vi "Ref_2_R.vi"(0 "Control  Ch 3":refnum<vi>, 1 "Control  Ch 4":refnum<vi>, 2 "Control  Ch 5":refnum<vi>, 3 "Init_F":bool=TRUE, 4 "Control  Ch 6":refnum<vi>, 5 "Control  Ch 7":refnum<vi>, 6 "Control  Ch 8":refnum<vi>, 7 "error in":errorcluster, 8 "Control  Ch 2":refnum<vi>, 9 "Control  Ch 10":refnum<vi>, 10 "Control  Ch 1":refnum<vi>, 11 "Control  Ch 11":refnum<vi>, 12 "Control  Ch 9":refnum<vi>, 13 "Control  Ch 12":refnum<vi>) -> (15 "Control  Ch 12 out":refnum<vi>, 16 "Control  Ch 10 out":refnum<vi>, 17 "Control  Ch 1 out":refnum<vi>, 18 "Control  Ch 9 out":refnum<vi>, 19 "Control  Ch 2 out":refnum<vi>, 20 "Control  Ch 11 out":refnum<vi>, 21 "Control  Ch 8 out":refnum<vi>, 22 "Control  Ch 7 out":refnum<vi>, 23 "Control  Ch 6 out":refnum<vi>, 24 "Control  Ch 5 out":refnum<vi>, 25 "Control  Ch 4 out":refnum<vi>, 26 "Control  Ch 3 out":refnum<vi>, 27 "error out":errorcluster)   [LabVIEW 2017]
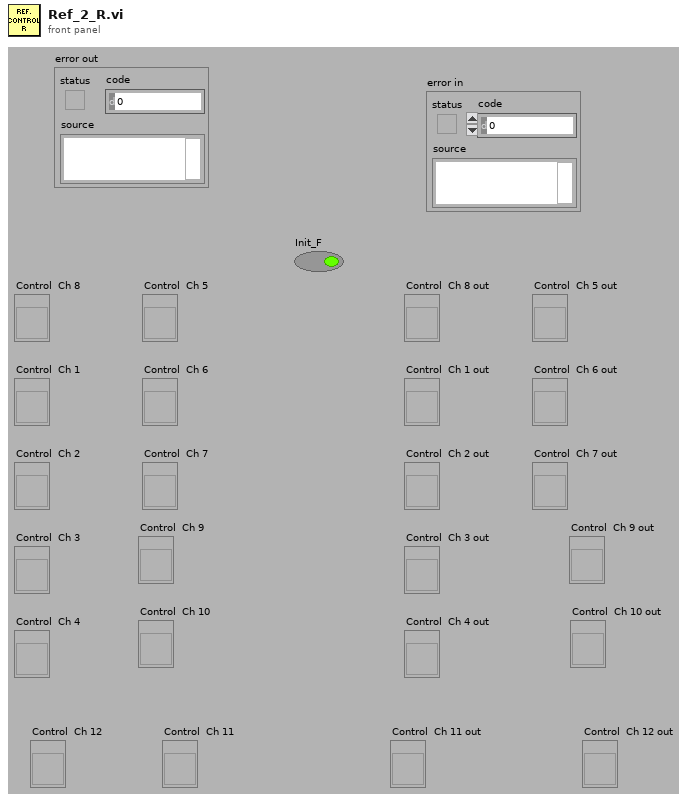
[diagram p1: front panel]
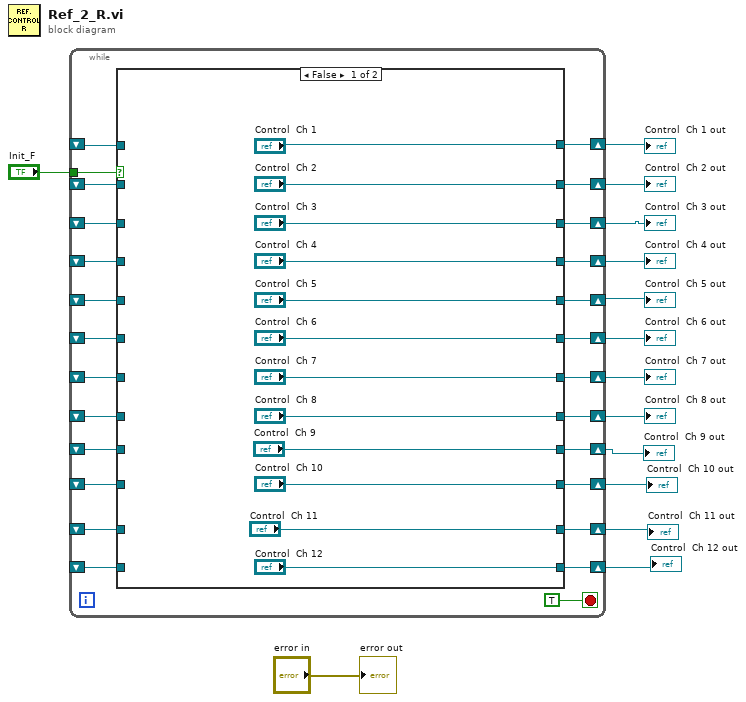
[diagram p0: block diagram]
diagram:
  n1 = while {
    shift-right: [w39] -> w12
    shift-left: _ -> [w38]
    tunnel: "Init_F" -> [w37]
    shift-right: [w36] -> w11
    shift-left: _ -> [w29]
    shift-right: [w35] -> w8
    shift-left: _ -> [w28]
    shift-right: [w34] -> w10
    shift-left: _ -> [w23]
    shift-right: [w33] -> w9
    shift-left: _ -> [w27]
    shift-right: [w32] -> w7
    shift-left: _ -> [w26]
    shift-right: [w31] -> w6
    shift-left: _ -> [w25]
    shift-right: [w30] -> w5
    shift-left: _ -> [w24]
    shift-right: [w22] -> w4
    shift-left: _ -> [w20]
    shift-right: [w21] -> w3
    shift-left: _ -> [w19]
    shift-right: [w18] -> w1
    shift-left: _ -> [w16]
    shift-right: [w17] -> w2
    shift-left: _ -> [w15]
    stop <- TRUE stop-if-true
    n2 = case shown="False" w37 {
      tunnel: ["Control  Ch 1" w64] -> w39
      tunnel: w38 -> [_ w64]
      tunnel: ["Control  Ch 2" w57] -> w36
      tunnel: ["Control  Ch 3" w58] -> w35
      tunnel: ["Control  Ch 4" w59] -> w34
      tunnel: ["Control  Ch 5" w60] -> w33
      tunnel: ["Control  Ch 6" w61] -> w32
      tunnel: ["Control  Ch 7" w62] -> w31
      tunnel: ["Control  Ch 8" w63] -> w30
      tunnel: w29 -> [_ w57]
      tunnel: w28 -> [_ w58]
      tunnel: w27 -> [_ w60]
      tunnel: w26 -> [_ w61]
      tunnel: w25 -> [_ w62]
      tunnel: w24 -> [_ w63]
      tunnel: w23 -> [_ w59]
      tunnel: ["Control  Ch 9" w56] -> w22
      tunnel: ["Control  Ch 10" w55] -> w21
      tunnel: w20 -> [_ w56]
      tunnel: w19 -> [_ w55]
      tunnel: ["Control  Ch 11" w54] -> w18
      tunnel: ["Control  Ch 12" w53] -> w17
      tunnel: w16 -> [_ w54]
      tunnel: w15 -> [_ w53]
      frame False {
      }
      frame True {
      }
    }
  }
  "Control  Ch 8 out" <- w5
  "Control  Ch 7 out" <- w6
  "Control  Ch 6 out" <- w7
  "Control  Ch 5 out" <- w9
  "Control  Ch 4 out" <- w10
  "Control  Ch 3 out" <- w8
  "Control  Ch 2 out" <- w11
  "Control  Ch 1 out" <- w12
  "Control  Ch 9 out" <- w4
  "Control  Ch 10 out" <- w3
  "Control  Ch 11 out" <- w1
  "Control  Ch 12 out" <- w2
  "error out" <- "error in"
